vi "Get Options from DVR.vi"(8 "Error In":errorcluster, 11 "Options DVR":T2) -> (0 "Error Out":errorcluster, 2 "Options":T1, 3 "Options DVR":T2)   [LabVIEW 2011]
uses:
  Controls/Options DVR.ctl
  Controls/Options.ctl
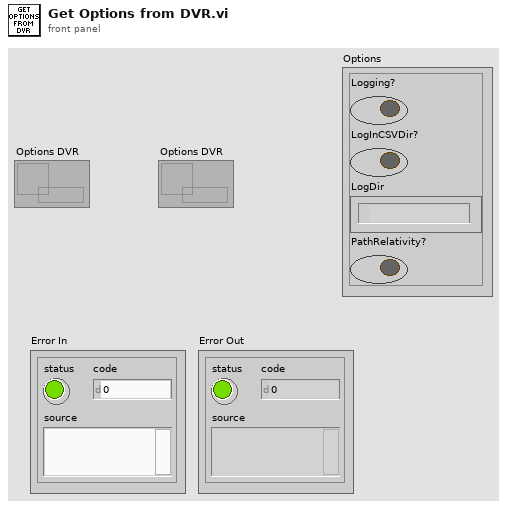
[diagram p1: front panel]
types:
  T1 = typedef "Options.ctl" = cluster{"Logging?":bool, "LogInCSVDir?":bool, "LogDir":path, "PathRelativity?":bool}
  T2 = typedef "Options DVR.ctl" = refnum<data-value>
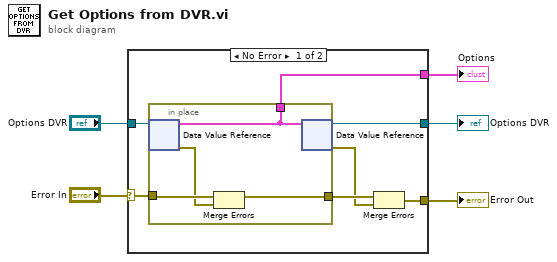
[diagram p0: block diagram]
diagram:
  n1 = case shown="No Error" "Error In" {
    selector: "Error In" -> [w6 w18]
    tunnel: "Options DVR" -> [w12 w17]
    tunnel: [w9 _] -> w4
    tunnel: [w8 w18] -> w3
    tunnel: [w7 w17] -> w2
    frame No Error {
      n2 = in-place {
        in-place-border: w6 -> [w16]
        in-place-border: [w14] -> w11
        in-place-border: [w13] -> w9
        n3 = in-place-dvr #1(w12) -> (w13:T1, w15:errorcluster)
        n4 = Merge Errors(w16, w15) -> (w14:errorcluster)
        n5 = in-place-dvr #1(w13) -> (w7:T2, w10:errorcluster)
      }
      n6 = Merge Errors(w11, w10) -> (w8:errorcluster)
    }
    frame Error {
    }
  }
  "Error Out" <- w3
  "Options DVR" <- w2
  "Options" <- w4
